vi "FrameChart.vi"(9 "Frame IN":u8[](array[numeric]), 10 "Frame NAK":u8[](array[numeric]), 11 "Frame Out":u8[](array[numeric])) -> (2 "CountOfTransactionsInFrame":i32, 3 "Frame":cluster{i32[], i32[]}[](graph))   [LabVIEW 2014]
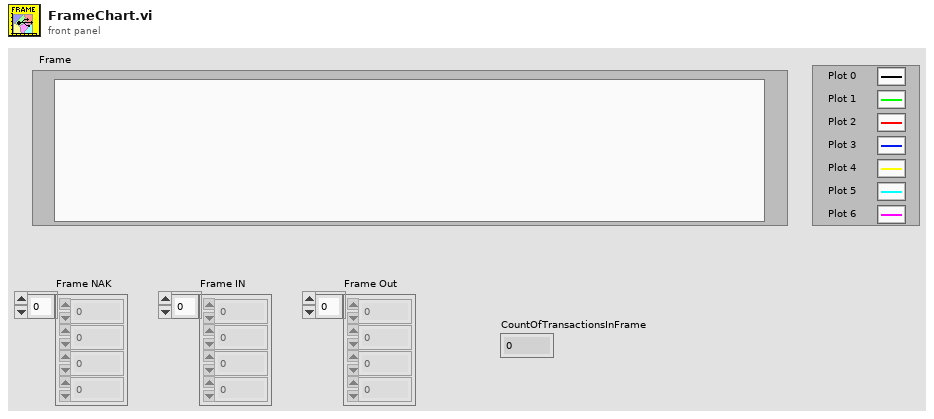
[diagram p1: front panel]
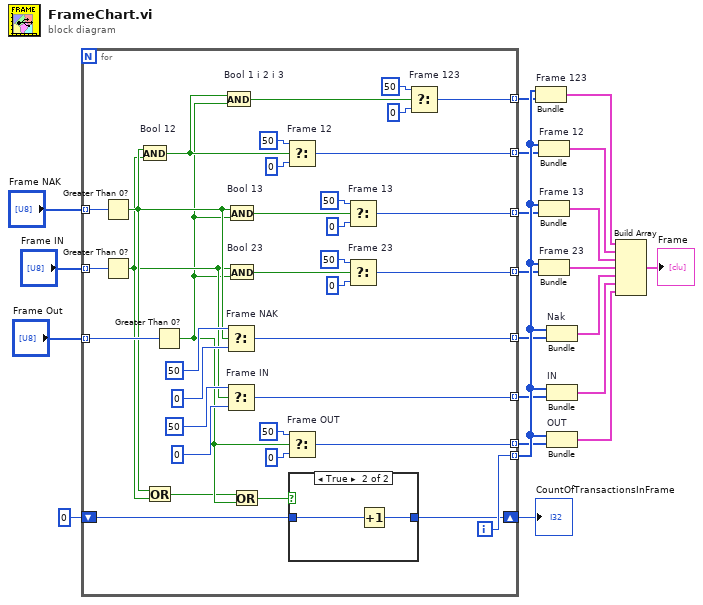
[diagram p0: block diagram]
diagram:
  n1 = for {
    tunnel: "Frame NAK" -> [w32] mode=indexing
    tunnel: "Frame IN" -> [w31] mode=indexing
    tunnel: "Frame Out" -> [w30] mode=indexing
    tunnel: [w40] -> w10 mode=indexing
    tunnel: [w39] -> w9 mode=indexing
    tunnel: [w38] -> w8 mode=indexing
    tunnel: [w37] -> w7 mode=indexing
    tunnel: [w36] -> w6 mode=indexing
    tunnel: [w35] -> w5 mode=indexing
    tunnel: [w34] -> w4 mode=indexing
    tunnel: [w33] -> w3 mode=indexing
    shift-right: [w27] -> w1
    shift-left: 0 -> [w28]
    i -> [w40]
    n2 = Greater Than 0?(x=w32) -> (x > 0?=w26:bool)
    n3 = Greater Than 0?(x=w31) -> (x > 0?=w25:bool)
    n4 = And "Bool 12"(x=w26, y=w25) -> (x .and. y?=w43:bool)
    n5 = Or(x=w26, y=w25) -> (x .or. y?=w23:bool)
    n6 = Greater Than 0?(x=w30) -> (x > 0?=w24:bool)
    n7 = And "Bool 1 i 2 i 3"(x=w43, y=w24) -> (x .and. y?=w29:bool)
    n8 = Select "Frame NAK"(t=50, s=w26, f=0) -> (s? t:f=w35:i32)
    n9 = Select "Frame IN"(t=50, s=w25, f=0) -> (s? t:f=w34:i32)
    n10 = And "Bool 13"(x=w26, y=w24) -> (x .and. y?=w42:bool)
    n11 = And "Bool 23"(x=w25, y=w24) -> (x .and. y?=w41:bool)
    n12 = Or(x=w23, y=w24) -> (x .or. y?=w22:bool)
    n13 = Select "Frame 12"(t=50, s=w43, f=0) -> (s? t:f=w38:i32)
    n14 = Select "Frame OUT"(t=50, s=w24, f=0) -> (s? t:f=w33:i32)
    n15 = case shown="True" w22 {
      tunnel: w28 -> [w58 w60]
      tunnel: [w58 w59] -> w27
      frame False {
      }
      frame True {
        n16 = Increment(x=w60) -> (x+1=w59:i32)
      }
    }
    n17 = Select "Frame 13"(t=50, s=w42, f=0) -> (s? t:f=w37:i32)
    n18 = Select "Frame 23"(t=50, s=w41, f=0) -> (s? t:f=w36:i32)
    n19 = Select "Frame 123"(t=50, s=w29, f=0) -> (s? t:f=w39:i32)
  }
  "CountOfTransactionsInFrame" <- w1
  n20 = Bundle "Frame 123"(w10, w9) -> (w17:cluster{i32[], i32[]})  [unwired: 1 in]
  n21 = Bundle "Frame 12"(w10, w8) -> (w16:cluster{i32[], i32[]})  [unwired: 1 in]
  n22 = Bundle "Frame 13"(w10, w7) -> (w15:cluster{i32[], i32[]})  [unwired: 1 in]
  n23 = Bundle "Frame 23"(w10, w6) -> (w14:cluster{i32[], i32[]})  [unwired: 1 in]
  n24 = Bundle "Nak"(w10, w5) -> (w13:cluster{i32[], i32[]})  [unwired: 1 in]
  n25 = Bundle "IN"(w10, w4) -> (w12:cluster{i32[], i32[]})  [unwired: 1 in]
  n26 = Bundle "OUT"(w10, w3) -> (w11:cluster{i32[], i32[]})  [unwired: 1 in]
  n27 = Build Array(w17, w16, w15, w14, w13, w12, w11) -> (→"Frame":cluster{i32[], i32[]}[])
